vi "Read from Inline Execution Units.vi"(8 "error in (no error)":errorcluster, 11 "RTStateVariables in":T1 {"Inline Execution Units"."Outgoing Data References"."Data Reference" format="%.0x"; "Inline Execution Units"."Incoming Data References" format="%.0x"}) -> (0 "error out":errorcluster, 3 "RTStateVariables out":T1 {"Inline Execution Units"."Outgoing Data References"."Data Reference" format="%.0x"; "Inline Execution Units"."Incoming Data References" format="%.0x"})   [LabVIEW 2020, in "Ballard ARINC 429 Engine.lvlib" / "Custom Device.lvlib"]
uses:
  Custom Device.lvlib
  RTStateVariables.ctl
  <vilib>/NI/NIVS Inline Async API/_VS Inline Async API/VS Inline Async API/VS Inline Async API.lvclass
  Interfaces/Shared Resources/Shared Resources.lvclass
  Inline Execution Unit Runtime Information.ctl
  Interfaces/Execution Unit/Execution Unit.lvclass
  <vilib>/NI VeriStand/Custom Device API/Data Reference.ctl
  <vilib>/NI VeriStand/Custom Device API/Block Data Reference.ctl
  Asynchronous Execution Unit Runtime Information.ctl
  <vilib>/NI VeriStand/Custom Device API/Global Data Refs.vi
  <vilib>/NI VeriStand/Custom Device API/Custom Device API.lvlib
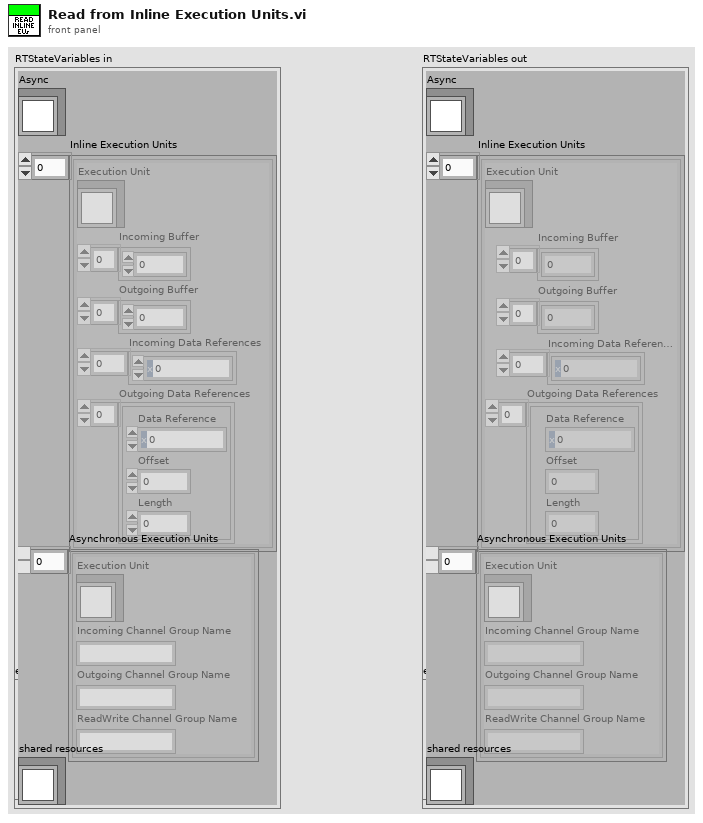
[diagram p1: front panel]
types:
  T1 = typedef "Ballard ARINC 429 Engine.lvlib/Custom Device.lvlib/RTStateVariables.ctl" = cluster{"Async":refnum<class "VS Inline Async API.lvclass">, "Inline Execution Units":T2[], "Asynchronous Execution Units":T5[], "shared resources":refnum<class "Shared Resources.lvclass">}
  T2 = typedef "Ballard ARINC 429 Engine.lvlib/Custom Device.lvlib/Inline Execution Unit Runtime Information.ctl" = cluster{"Execution Unit":refnum<class "Execution Unit.lvclass">, "Incoming Buffer":dbl[], "Outgoing Buffer":dbl[], "Incoming Data References":T3[], "Outgoing Data References":T4[]}
  T3 = typedef "Custom Device API.lvlib/Data Reference.ctl" = i32
  T4 = typedef "Custom Device API.lvlib/Block Data Reference.ctl" = cluster{"Data Reference":T3, "Offset":u64, "Length":u64}
  T5 = typedef "Ballard ARINC 429 Engine.lvlib/Custom Device.lvlib/Asynchronous Execution Unit Runtime Information.ctl" = cluster{"Execution Unit":refnum<class "Execution Unit.lvclass">, "Incoming Channel Group Name":string, "Outgoing Channel Group Name":string, "ReadWrite Channel Group Name":string}
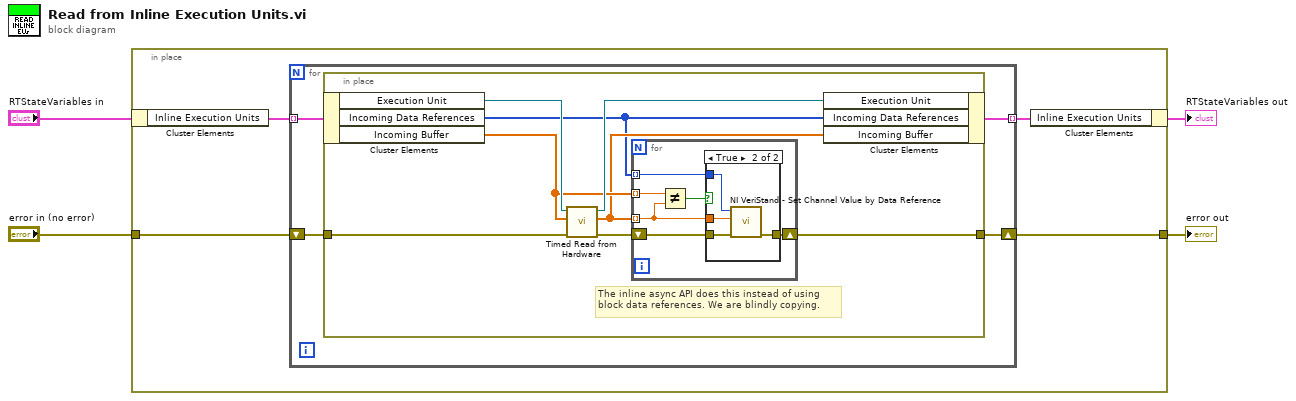
[diagram p0: block diagram]
diagram:
  n1 = in-place {
    in-place-border: [w8] -> w4
    in-place-border: "error in (no error)" -> [w7]
    n2 = in-place-cluster #1("RTStateVariables in") -> ("Inline Execution Units"=w6:T2[])
    n3 = for {
      tunnel: [w10] -> w5 mode=indexing
      tunnel: w6 -> [w9] mode=indexing
      shift-right: [w12] -> w8
      shift-left: w7 -> [w11]
      n4 = in-place {
        in-place-border: w11 -> [w18]
        in-place-border: [w14] -> w12
        # "The inline async API does this instead of using\nblock data references. We are blindly copying."
        n5 = in-place-cluster #2(w9) -> ("Execution Unit"=w20:refnum<class "Execution Unit.lvclass">, "Incoming Data References"=w13:T3[], "Incoming Buffer"=w17:dbl[])
        n6 = call "Timed Read from Hardware.vi"("error in"=w18, "Values in"=w17, "Execution Unit in"=w20) -> ("error out"=w15:errorcluster, "Values out"=w16:dbl[], "Execution Unit out"=w19:refnum<class "Execution Unit.lvclass">)  [unwired: 6 in]
        n7 = for {
          tunnel: w17 -> [w23] mode=indexing
          tunnel: w16 -> [w22] mode=indexing
          shift-right: [w24] -> w14
          shift-left: w15 -> [w25]
          tunnel: w13 -> [w21] mode=indexing
          n8 = Not Equal?(x=w23, y=w22) -> (x != y?=w26:bool)
          n9 = case shown="True" w26 {
            tunnel: w25 -> [w27 w31]
            tunnel: [w27 w30] -> w24
            tunnel: w22 -> [_ w29]
            tunnel: w21 -> [_ w28]
            frame False {
            }
            frame True {
              n10 = call <vilib>:"NI VeriStand - Set Channel Value by Data Reference.vi"("error in (no error)"=w31, "Value"=w29, "Data Reference in"=w28) -> ("error out"=w30:errorcluster)  [unwired: 8 in]
            }
          }
        }
        n11 = in-place-cluster #2("Execution Unit"=w19, "Incoming Data References"=w13, "Incoming Buffer"=w16) -> (w10:T2)
      }
    }
    n12 = in-place-cluster #1("Inline Execution Units"=w5) -> (→"RTStateVariables out":T1)
  }
  "error out" <- w4
